vi "textParse.vi"(8 "error in (no error)":errorcluster, 10 "file name":string, 11 "base path":path=path "C:/Users/bryan.lee/Desktop/Specification sheets") -> (0 "error out":errorcluster, 2 "all rows":string[][](array[string]), 3 "appended path":path)   [LabVIEW 2018]
uses:
  <vilib>/Utility/file.llb/Read Delimited Spreadsheet (string).vi
panel:
  out "element 30":string
  out "element 29":string
  out "element 28":string
  out "Foldback (set max":string
  out "Foldback (set min":string
  out "Current low limit Max":string
  out "Current low limit Min":string
  out "Current high limit Max":string
  out "Current high limit Min":string
  out "IRcomp (set Max":string
  out "IRcomp (set min":string
  out "Speed pot min":string
  out "FET driver PWM max":string
  out "FET driver PWM min":string
  out "HV Bus":string
  out "V Max Rated":string
  out "V Rated Output":string
  out "Ripple/Noise max":string
  out "Ripple/Noise min":string
  out "Voltage drift Max":string
  out "Voltage drift Min":string
  out "Voltage Output":string
  out "Input Allowable":string
  out "Input Current":string
  out "Input Voltage":string
  out "Vendor Number":string
  out "Vendor Name":string
  out "Firmware":string
  out "Part Number":string
  out "Part Name":string
  # "Global variables"
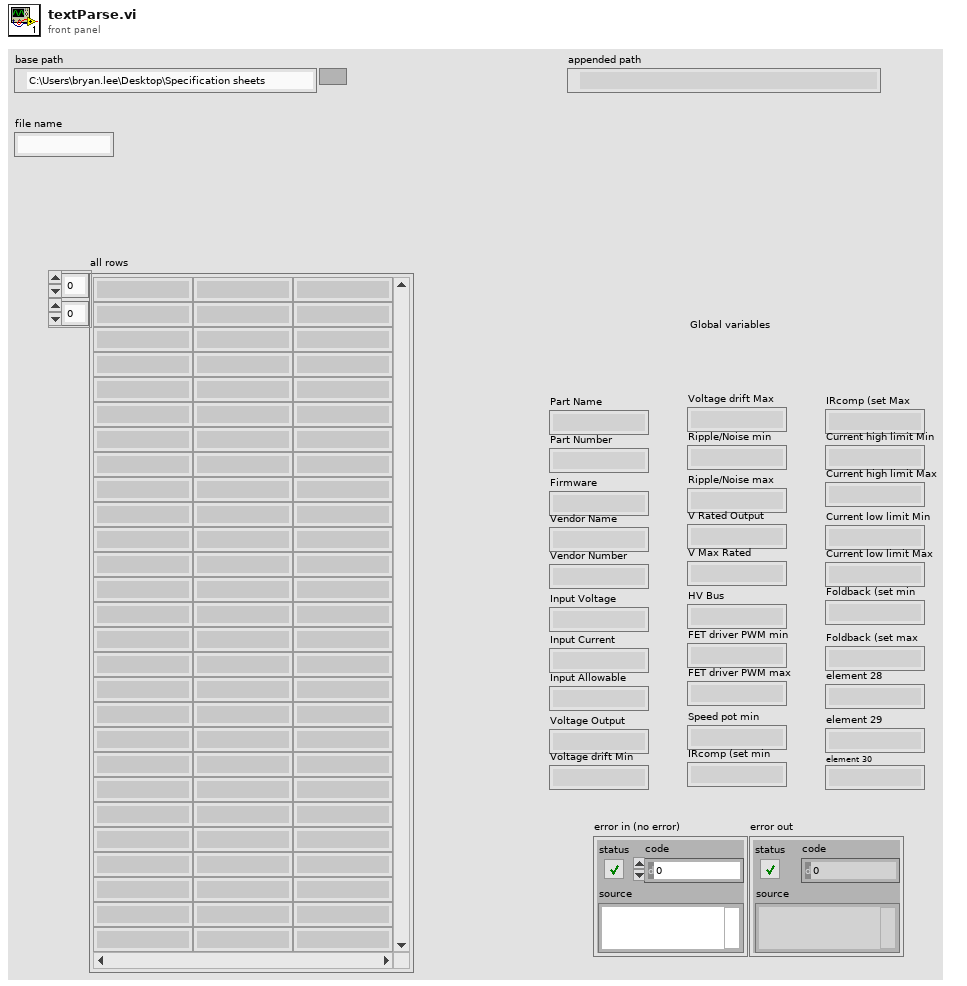
[diagram p1: front panel]
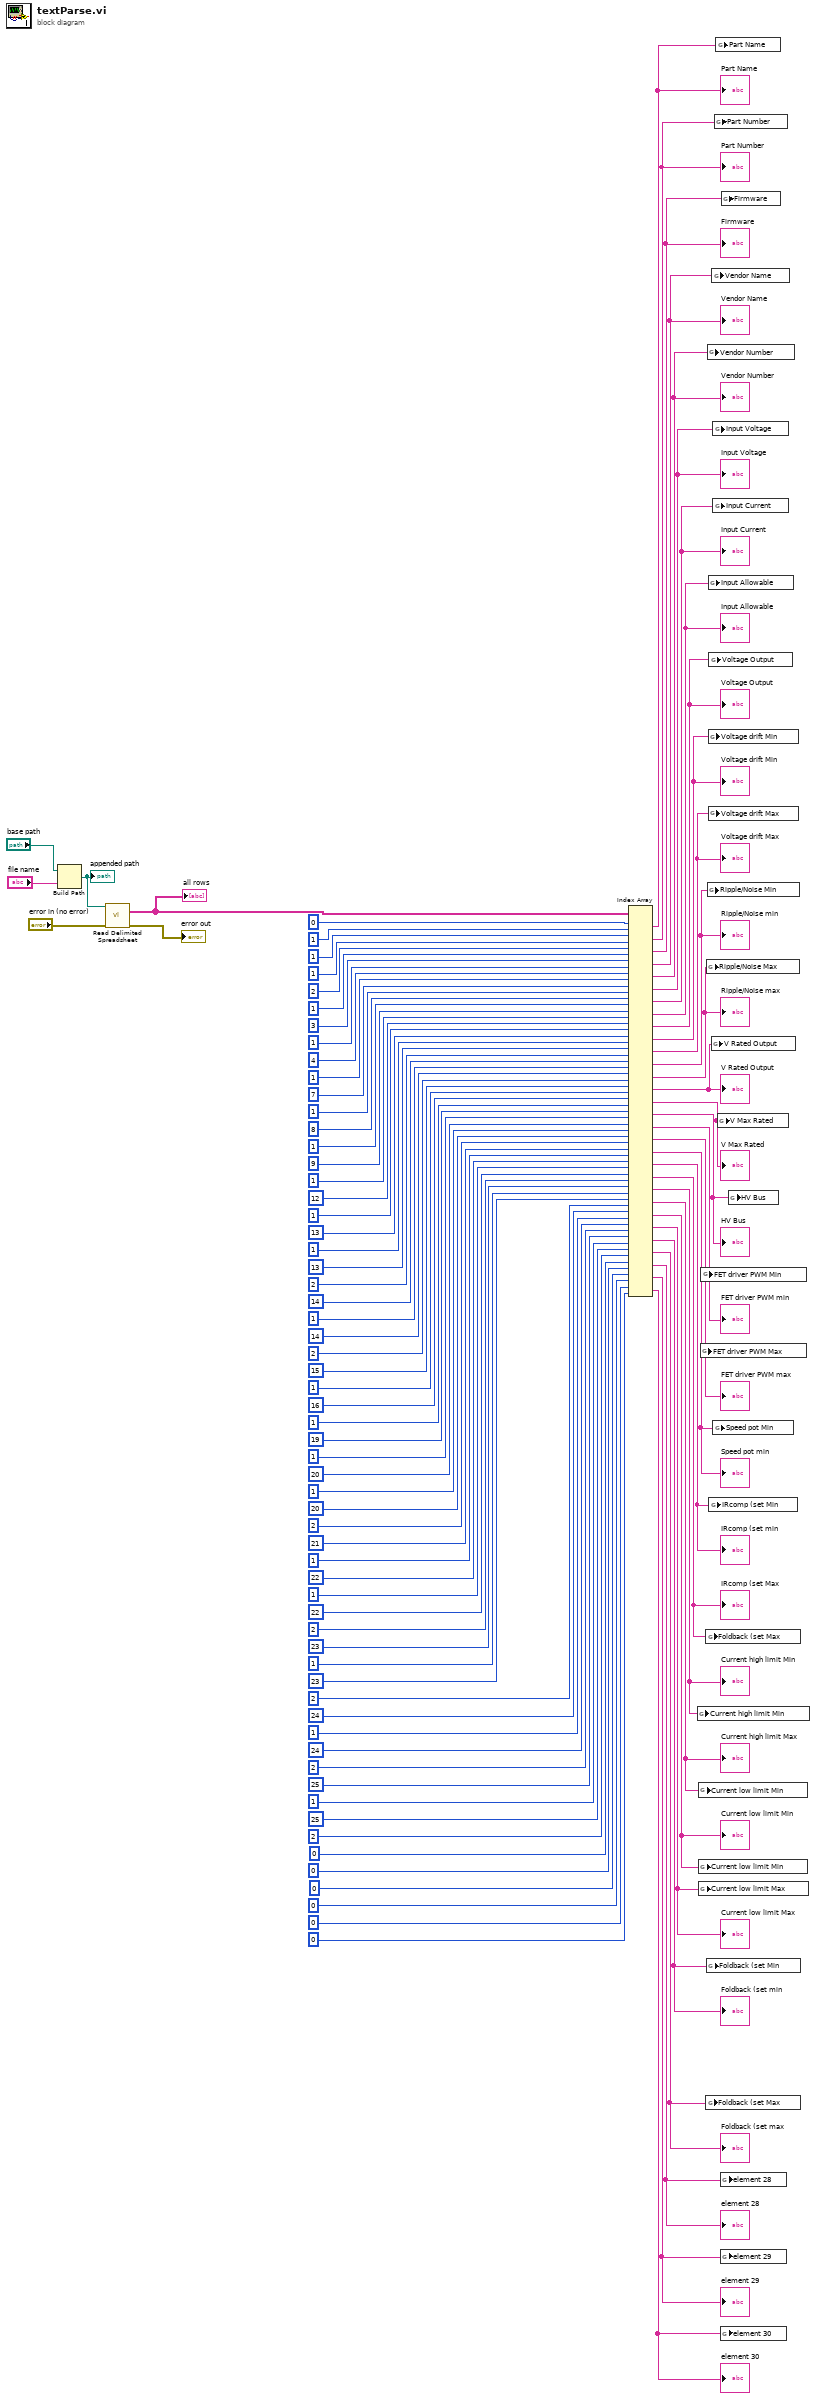
[diagram p0: block diagram]
diagram:
  n1 = Build Path(base path="base path", name or relative path="file name") -> (appended path=w3:path)
  "appended path" <- w3
  n2 = call-poly <vilib>:"Read Delimited Spreadsheet.vi"("file path (dialog if empty)"=w3, "error in (no error)"="error in (no error)") -> ("all rows"=w4:string[][], "error out"=→"error out":errorcluster)  [unwired: 8 in, 4 out]
  "all rows" <- w4
  n3 = Index Array(array=w4, index (row) #1=0 ("index (row)"), index (col) #1=1 ("disabled index (col)"), index (row) #2=1 ("index (row) 2"), index (col) #2=1 ("disabled index (col) 2"), index (row) #3=2 ("index (row) 3"), index (col) #3=1 ("disabled index (col) 3"), index (row) #4=3 ("index (row) 4"), index (col) #4=1 ("disabled index (col) 4"), index (row) #5=4 ("index (row) 5"), index (col) #5=1 ("disabled index (col) 5"), index (row) #6=7 ("index (row) 6"), index (col) #6=1 ("disabled index (col) 6"), index (row) #7=8 ("index (row) 7"), index (col) #7=1 ("disabled index (col) 7"), index (row) #8=9 ("index (row) 8"), index (col) #8=1 ("disabled index (col) 8"), index (row) #9=12 ("index (row) 9"), index (col) #9=1 ("disabled index (col) 9"), index (row) #10=13 ("index (row) 10"), index (col) #10=1 ("disabled index (col) 10"), index (row) #11=13 ("index (row) 11"), index (col) #11=2 ("disabled index (col) 11"), index (row) #12=14 ("index (row) 12"), index (col) #12=1 ("disabled index (col) 12"), index (row) #13=14 ("index (row) 13"), index (col) #13=2 ("disabled index (col) 13"), index (row) #14=15 ("index (row) 14"), index (col) #14=1 ("disabled index (col) 14"), index (row) #15=16 ("index (row) 15"), index (col) #15=1 ("disabled index (col) 15"), index (row) #16=19 ("index (row) 16"), index (col) #16=1 ("disabled index (col) 16"), index (row) #17=20 ("index (row) 17"), index (col) #17=1 ("disabled index (col) 17"), index (row) #18=20 ("index (row) 18"), index (col) #18=2 ("disabled index (col) 18"), index (row) #19=21 ("index (row) 19"), index (col) #19=1 ("disabled index (col) 19"), index (row) #20=22 ("index (row) 20"), index (col) #20=1 ("disabled index (col) 20"), index (row) #21=22 ("index (row) 21"), index (col) #21=2 ("disabled index (col) 21"), index (row) #22=23 ("index (row) 22"), index (col) #22=1 ("disabled index (col) 22"), index (row) #23=23 ("index (row) 23"), index (col) #23=2 ("disabled index (col) 23"), index (row) #24=24 ("index (row) 24"), index (col) #24=1 ("disabled index (col) 24"), index (row) #25=24 ("index (row) 25"), index (col) #25=2 ("disabled index (col) 25"), index (row) #26=25 ("index (row) 26"), index (col) #26=1 ("disabled index (col) 26"), index (row) #27=25 ("index (row) 27"), index (col) #27=2 ("disabled index (col) 27"), index (row) #28=0 ("index (row) 28"), index (col) #28=0 ("disabled index (col) 28"), index (row) #29=0 ("index (row) 29"), index (col) #29=0 ("disabled index (col) 29"), index (row) #30=0 ("index (row) 30"), index (col) #30=0 ("disabled index (col) 30")) -> (element #1=w76:string, element #2=w75:string, element #3=w74:string, element #4=w73:string, element #5=w72:string, element #6=w71:string, element #7=w70:string, element #8=w69:string, element #9=w68:string, element #10=w67:string, element #11=w26:string, element #12=w25:string, element #13=w24:string, element #14=w23:string, element #15=w22:string, element #16=w21:string, element #17=w20:string, element #18=w19:string, element #19=w18:string, element #20=w17:string, element #21=w16:string, element #22=w15:string, element #23=w14:string, element #24=w7:string, element #25=w13:string, element #26=w12:string, element #27=w11:string, element #28=w10:string, element #29=w9:string, element #30=w8:string)
  "Part Name" <- w76
  "Part Number" <- w75
  "Firmware" <- w74
  "Vendor Name" <- w73
  "Vendor Number" <- w72
  "Input Voltage" <- w71
  "Input Current" <- w70
  "Input Allowable" <- w69
  "Voltage Output" <- w68
  "Voltage drift Min" <- w67
  "Voltage drift Max" <- w26
  "Ripple/Noise min" <- w25
  "Ripple/Noise max" <- w24
  "V Rated Output" <- w23
  "V Max Rated" <- w22
  "HV Bus" <- w21
  "FET driver PWM min" <- w20
  "FET driver PWM max" <- w19
  "Speed pot min" <- w18
  "IRcomp (set min" <- w17
  "IRcomp (set Max" <- w16
  "Current high limit Min" <- w15
  "Current high limit Max" <- w14
  "Current low limit Min" <- w7
  "Current low limit Max" <- w13
  "Foldback (set min" <- w12
  "Foldback (set max" <- w11
  "element 28" <- w10
  "element 29" <- w9
  "element 30" <- w8
  n4 = global write "Global textParse.vi" "Current high limit Min"(w15) -> ()
  n5 = global write "Global textParse.vi" "Current low limit Min"(w14) -> ()
  n6 = global write "Global textParse.vi" "Current low limit Min"(w7) -> ()
  n7 = global write "Global textParse.vi" "Current low limit Max"(w13) -> ()
  n8 = global write "Global textParse.vi" "FET driver PWM Max"(w19) -> ()
  n9 = global write "Global textParse.vi" "FET driver PWM Min"(w20) -> ()
  n10 = global write "Global textParse.vi" "Foldback (set Max"(w16) -> ()
  n11 = global write "Global textParse.vi" "Foldback (set Max"(w11) -> ()
  n12 = global write "Global textParse.vi" "Ripple/Noise Max"(w24) -> ()
  n13 = global write "Global textParse.vi" "Foldback (set Min"(w12) -> ()
  n14 = global write "Global textParse.vi" "Vendor Number"(w72) -> ()
  n15 = global write "Global textParse.vi" "Ripple/Noise Min"(w25) -> ()
  n16 = global write "Global textParse.vi" "Input Allowable"(w69) -> ()
  n17 = global write "Global textParse.vi" "Voltage drift Min"(w67) -> ()
  n18 = global write "Global textParse.vi" "Voltage drift Max"(w26) -> ()
  n19 = global write "Global textParse.vi" "Voltage Output"(w68) -> ()
  n20 = global write "Global textParse.vi" "IRcomp (set Min"(w17) -> ()
  n21 = global write "Global textParse.vi" "V Rated Output"(w23) -> ()
  n22 = global write "Global textParse.vi" "Vendor Name"(w73) -> ()
  n23 = global write "Global textParse.vi" "Input Voltage"(w71) -> ()
  n24 = global write "Global textParse.vi" "Input Current"(w70) -> ()
  n25 = global write "Global textParse.vi" "Speed pot Min"(w18) -> ()
  n26 = global write "Global textParse.vi" "Part Number"(w75) -> ()
  n27 = global write "Global textParse.vi" "Part Name"(w76) -> ()
  n28 = global write "Global textParse.vi" "V Max Rated"(w22) -> ()
  n29 = global write "Global textParse.vi" "element 28"(w10) -> ()
  n30 = global write "Global textParse.vi" "element 29"(w9) -> ()
  n31 = global write "Global textParse.vi" "element 30"(w8) -> ()
  n32 = global write "Global textParse.vi" "Firmware"(w74) -> ()
  n33 = global write "Global textParse.vi" "HV Bus"(w21) -> ()
